vi "ResonanceAnalyzer.vi"() -> ()   [LabVIEW 2014]
doc: "This VI reads a spreadsheet .txt data file of the Kundt's tube and then performs a curve fit reports the RMS amplitude at resonance, the resonant frequency, and the Q factor. The VI can also simulate a data set with supplied parameters, add guassian noise and verify the fit worls correctly. This simulated data can also be used to adjust the best guess to fit parameters."
uses:
  <vilib>/imath/engines/lvmath2/RunTimeEngine/Managers/WorkSpace/UID Generator.vi
  <vilib>/imath/engines/lvmath2/RunTimeEngine/RangeToken/NIMS_Range.vi
  <instcachedir>/0/NIMS_Range_9BCE657718DF4976A877346C61F22738.lvgen/NIMS_Range_9BCE657718DF4976A877346C61F22738_000.vi
  <vilib>/imath/engines/lvmath2/RunTimeEngine/RunTimeType/NIMS_RunTimeType_From StrictType (excl LVString).vi
  <instcachedir>/0/NIMS_RunTimeType_From StrictType (excl LVString)_15A5391EEA9C4AACB9955AC755B83D29.lvgen/NIMS_RunTimeType_From StrictType (excl LVString)_15A5391EEA9C4AACB9955AC755B83D29_000.vi
  <vilib>/imathl/engines/lvmath/Functions/Error Handling/Create Error.vi
  <vilib>/imath/engines/lvmath2/RunTimeEngine/LocalVariableDefStatement/MC_LocalVariableDefStatement_Display.vi
  <vilib>/imath/engines/lvmath2/RunTimeEngine/BuiltInFunctions/randnormal/NIMS_randnormal(1,I32).vi
  <vilib>/imath/engines/lvmath2/RunTimeEngine/ErrorHandling/NIMS_Error From Error Code.vi
  <vilib>/imath/engines/lvmath2/RunTimeEngine/ArithmeticOperatorToken/NIMS_ArithmeticOperator_minus.vi
  <instcachedir>/0/NIMS_ArithmeticOperator_minus_39C0593E74DA4138ACA2AB742906488D.lvgen/NIMS_ArithmeticOperator_minus_39C0593E74DA4138ACA2AB742906488D_003.vi
  <vilib>/imath/engines/lvmath2/RunTimeEngine/ArithmeticOperatorToken/NIMS_ArithmeticOperator_plus.vi
  <instcachedir>/0/NIMS_ArithmeticOperator_plus_48D6EAACA5D645B09F7EC9C016C2DEA8.lvgen/NIMS_ArithmeticOperator_plus_48D6EAACA5D645B09F7EC9C016C2DEA8_001.vi
  <vilib>/imath/engines/lvmath2/RunTimeEngine/Managers/SymbolTable/Clear UID.vi
  <vilib>/imath/engines/lvmath2/RunTimeEngine/NodeEndStatement/NIMS_NodeEndStatement_Output.vi
  <instcachedir>/0/NIMS_NodeEndStatement_Output_53EC0D466D134D7ABD903AC30B43404B.lvgen/NIMS_NodeEndStatement_Output_53EC0D466D134D7ABD903AC30B43404B_005.vi
  <instcachedir>/0/NIMS_NodeEndStatement_Output_53EC0D466D134D7ABD903AC30B43404B.lvgen/NIMS_NodeEndStatement_Output_53EC0D466D134D7ABD903AC30B43404B_000.vi
  <vilib>/imath/engines/lvmath2/RunTimeEngine/ErrorHandling/NIMS_Finalize Error.vi
  <vilib>/Utility/file.llb/Read From Spreadsheet File (DBL).vi
  <vilib>/imath/engines/lvmath2/RunTimeEngine/Managers/SymbolTable/NIMS_WorkSpace.lvlib
panel:
  out "XY Graph":cluster{"f":dbl[], "y":dbl[]}[](graph)=[{"f"=[600.0, 605.0, 610.0, 615.0, 620.0, 625.0, 630.0, 635.0, 640.0, 645.0, 650.0, 655.0, 660.0, 665.0, 670.0, 675.0, 680.0, 685.0, 690.0, 695.0, 700.0, 705.0, 710.0, 715.0, 720.0, 725.0, 730.0, 735.0, 740.0, 745.0, 750.0], "y"=[8.44455949876584e-06, 2.0687737645322164e-05, 2.1920805063266238e-05, 8.006459294470547e-06, 8.134127957802083e-06, 3.173525556127131e-05, 5.869444494651924e-05, 7.24783002866334e-05, 0.0003042443346803616, 0.000393990273081269, 0.0002738479536639696, 0.00013256061186339, 6.174602437108711e-05, 2.9064141550805892e-05, 1.3727232833499853e-05, 2.434876846781405e-05, 6.273790322954604e-06, 7.031832221730014e-06, 1.0632441453683285e-05, 1.544182050752434e-05, 1.0053724958847406e-05, 4.129671437997426e-06, 5.19729657721199e-06, 9.553455829917101e-06, 1.6863064454931353e-05, 1.4538044705199302e-05, 6.9420621907848364e-06, 5.324079110095673e-06, 1.1821511253807668e-05, 1.4906201923285234e-05, 2.0779375921000738e-05]}, {"f"=[600.0, 605.0, 610.0, 615.0, 620.0, 625.0, 630.0, 635.0, 640.0, 645.0, 650.0, 655.0, 660.0, 665.0, 670.0, 675.0, 680.0, 685.0, 690.0, 695.0, 700.0, 705.0, 710.0, 715.0, 720.0, 725.0, 730.0, 735.0, 740.0, 745.0, 750.0], "y"=[9.742309710510184e-06, 1.4284231698794693e-05, 2.0109407197046786e-05, 2.784705514604789e-05, 3.86124152252423e-05, 5.4577400738027664e-05, 8.055489587814648e-05, 0.0001293229240316874, 0.00024220982951154673, 0.0004131276489269914, 0.0002324038082839859, 0.00012697191328891842, 8.068389932793836e-05, 5.570910422405969e-05, 4.02354544072139e-05, 2.9744798714693002e-05, 2.2175682921622603e-05, 1.646122732489114e-05, 1.1995970388910695e-05, 8.411442968558235e-06, 5.470807430672622e-06, 3.015006580200107e-06, 9.33306732387207e-07, -8.537334431389628e-07, -2.404574130377459e-06, -3.7631847817844656e-06, -4.963267835268104e-06, -6.0310877020440426e-06, -6.987413906606278e-06, -7.848885724936917e-06, -8.628989631075326e-06]}]
  out "Center Frequency":dbl=644.835248994041
  out "Q Factor":dbl=86.37766019704621
  out "Amplitude":dbl=0.00043892476055634055
  in  "?":enum32{"Sim", "Data"}(tab)=enum."Data"
  in  "Input Parameters":T1={"Q Factor"=10.0, "Center Frequency"=600.0, "Start Frequency"=400.0, "End Frequency"=800.0, "dF"=5.0, "Noise Level"=0.01, "RMS Voltage Amplitude"=2.0}
  # "Will curve fit data from a spreadsheet\n.txt file"
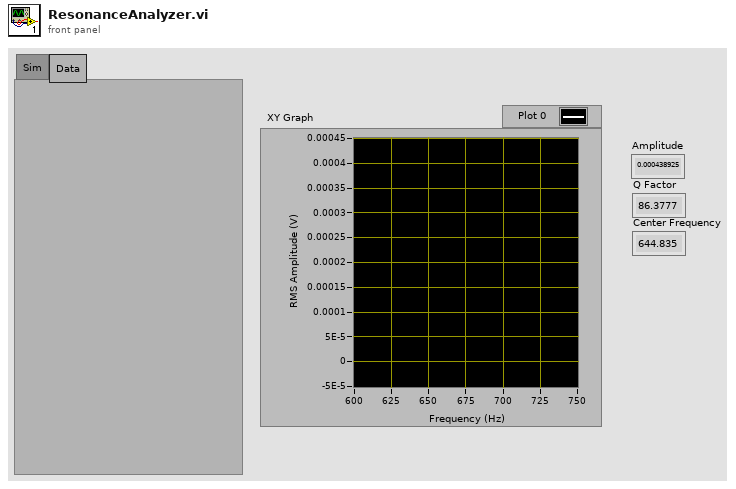
[diagram p1: front panel]
types:
  T1 = cluster{"Q Factor":dbl, "Center Frequency":dbl, "Start Frequency":dbl, "End Frequency":dbl, "dF":dbl, "Noise Level":dbl, "RMS Voltage Amplitude":dbl}
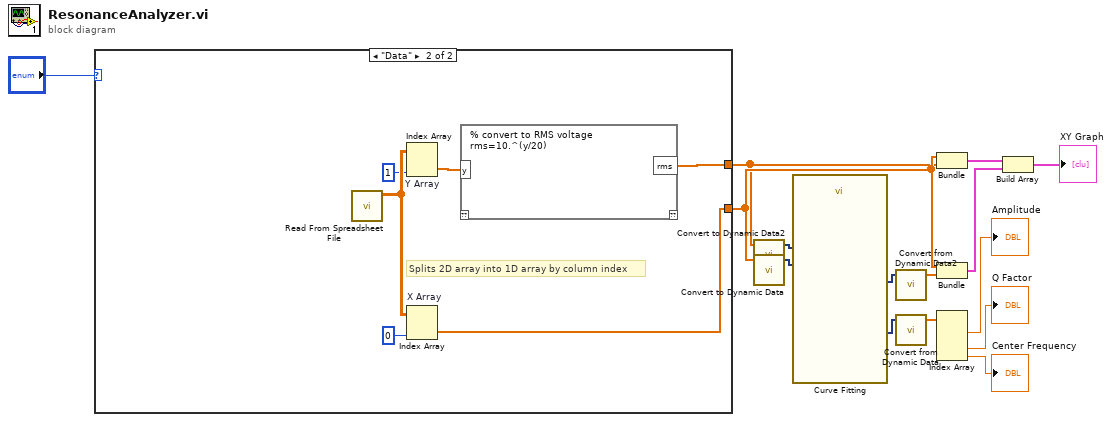
[diagram p0: block diagram]
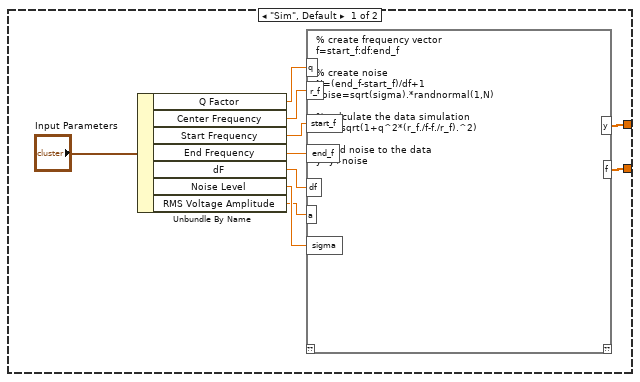
[diagram p2: hidden frame]
diagram:
  n1 = case shown="\"Data\"" "?" {
    tunnel: [w18 w200] -> w6
    tunnel: [w19 w201] -> w14
    frame "Sim", Default {
      n2 = Unbundle By Name("Input Parameters") -> ("Q Factor"=w24:dbl, "Center Frequency"=w23:dbl, "Start Frequency"=w22:dbl, "End Frequency"=w21:dbl, "dF"=w20:dbl, "Noise Level"=w17:dbl, "RMS Voltage Amplitude"=w16:dbl)
      n3 = mathscript code="% create frequency vector\nf=start_f:df:end_f\n\n% create noise\nN=(end_f-start_f)/df+1\nnoise=sqrt(sigma).*randnormal(1,N)\n\n% calculate the data simulation\ny=a./sqrt(1+q^2*(r_f./f-f./r_f).^2)\n\n% add noise to the data\ny=y+noise"("q"=w24, "r_f"=w23, "a"=w16, "df"=w20, "start_f"=w22, "end_f"=w21, "sigma"=w17) -> ("y"=w18:cdb[], "f"=w19:dbl[])  [unwired: 1 in, 1 out]
    }
    frame "Data" {
      # "Splits 2D array into 1D array by column index"
      n4 = call-poly <vilib>:"Read From Spreadsheet File.vi"() -> ("all rows"=w204:dbl[][])  [unwired: 7 in, 4 out]
      n5 = Index Array "Y Array"(array=w204, index (col)=1 ("disabled index (col)")) -> (element=w199:dbl[])  [unwired: 1 in]
      n6 = Index Array "X Array"(array=w204, index (col)=0 ("disabled index (col)")) -> (element=w201:dbl[])  [unwired: 1 in]
      n7 = mathscript code="% convert to RMS voltage\nrms=10.^(y/20)"("y"=w199) -> ("rms"=w200:dbl[])  [unwired: 1 in, 1 out]
    }
  }
  n8 = call "Convert to Dynamic Data2"("Array"=w6) -> ("Dynamic Data Type"=w12:dynamicdata)  [unwired: 3 in]
  n9 = call "Convert to Dynamic Data"("Array"=w14) -> ("Dynamic Data Type"=w13:dynamicdata)  [unwired: 3 in]
  n10 = call "Curve Fitting"("Locations"=w13, "Signals"=w12) -> ("best fit"=w8:dynamicdata, "non-linear coefficients"=w11:dynamicdata)  [unwired: 5 in, 3 out]
  n11 = call "Convert from Dynamic Data2"("Dynamic Data Type"=w8) -> ("Array"=w7:dbl[])  [unwired: 3 in]
  n12 = call "Convert from Dynamic Data"("Dynamic Data Type"=w11) -> ("Array"=w10:dbl[])  [unwired: 3 in]
  n13 = Bundle("all rows"=w14, "y"=w6) -> (w4:cluster{"all rows":dbl[], "y":cdb[]})  [unwired: 1 in]
  n14 = Bundle("all rows"=w14, "Array"=w7) -> (w5:cluster{"all rows":dbl[], "Array":dbl[]})  [unwired: 1 in]
  n15 = Index Array(array=w10) -> (element #1=→"Amplitude":dbl, element #3=→"Q Factor":dbl, element #4=→"Center Frequency":dbl)  [unwired: 4 in, 1 out]
  n16 = Build Array(w4, w5) -> (→"XY Graph":cluster{"all rows":dbl[], "y":cdb[]}[])
